vi "Layer2_TransmitAndReceiveResponse.vi"(4 "error in (no error)":errorcluster, 5 "Expecting Response":bool=TRUE, 6 "Message":string="TestStation1", 7 "Serial Port to Use":refnum<visa-resource-name>="COM8") -> (0 "Error Out":errorcluster, 1 "Response":string, 2 "Success":bool, 3 "Serial Port to Use (out)":refnum<visa-resource-name>)   [LabVIEW 2012]
uses:
  Arduino_Serial_GlobalConstants.vi
panel:
  out "Write Buffer":string
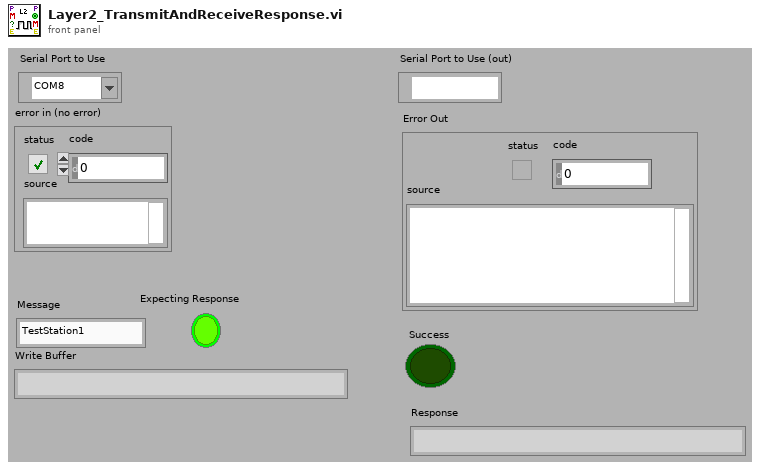
[diagram p1: front panel]
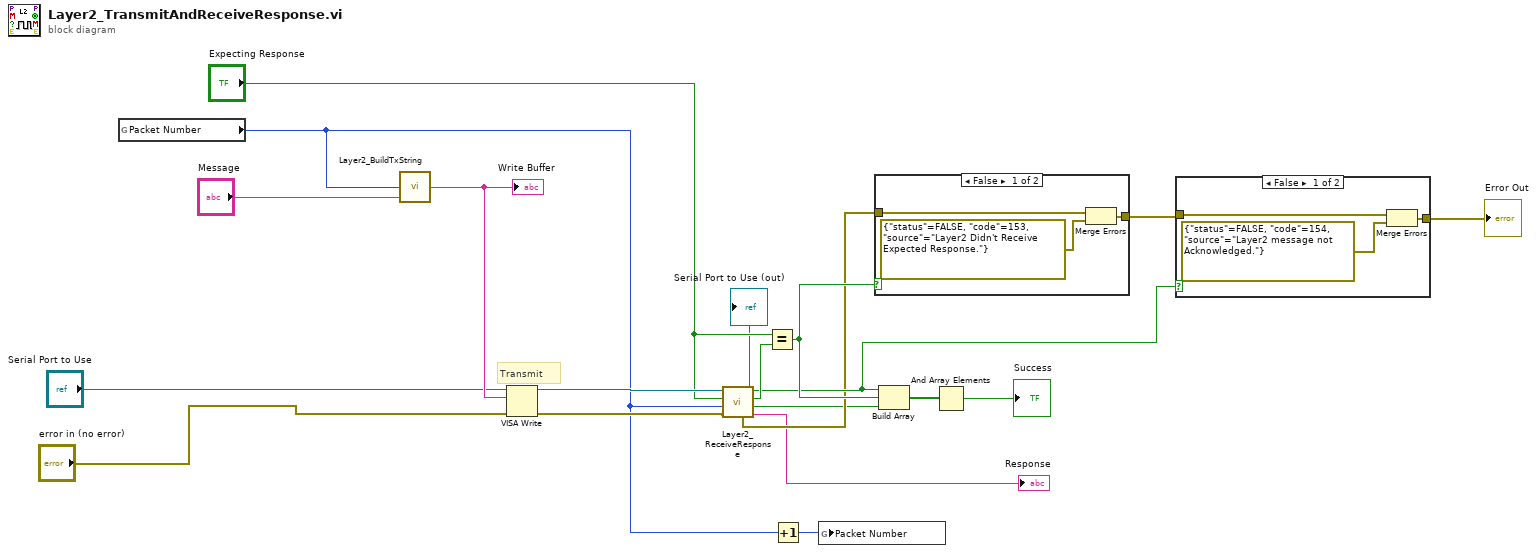
[diagram p0: block diagram]
diagram:
  # "Transmit"
  n1 = global read "Arduino_Serial_GlobalConstants.vi" "Packet Number"() -> (w11:u16)
  n2 = call "Layer2_BuildTxString.vi"("Message"="Message", "PacketNum"=w11) -> ("Write Buffer"=w17:string)  [unwired: 1 in]
  "Write Buffer" <- w17
  n3 = VISA Write(VISA resource name="Serial Port to Use", write buffer=w17, error in (no error)="error in (no error)") -> (VISA resource name out=w20:refnum<visa-resource-name>, error out=w19:errorcluster)  [unwired: 1 out]
  n4 = call "Layer2_ReceiveResponse.vi"("Error In"=w19, "PacketNum\nWaiting Ack"=w11, "Expecting Response"="Expecting Response", "Serial Port to Use"=w20) -> ("Layer2 Payload"=→"Response":string, "No Errors"=w5:bool, "Response Received"=w13:bool, "Msg Acknowledged"=w7:bool, "Error Out"=w6:errorcluster, "Serial Port to Use (out)"=→"Serial Port to Use (out)":refnum<visa-resource-name>)  [unwired: 2 in]
  n5 = Equal?(x="Expecting Response", y=w13) -> (x = y?=w10:bool)
  n6 = Increment(x=w11) -> (x+1=w14:u16)
  n7 = global write "Arduino_Serial_GlobalConstants.vi" "Packet Number"(w14) -> ()
  n8 = case shown="False" w10 {
    tunnel: w6 -> [w22 w24]
    tunnel: [w23 w24] -> w9
    frame False {
      n9 = Merge Errors(w22, errorcluster {"status"=FALSE, "code"=153, "source"="Layer2 Didn't Receive Expected Response."} ("error in")) -> (w23:errorcluster)
    }
    frame True {
    }
  }
  n10 = Build Array(w7, w10, w5) -> (w16:bool[])
  n11 = And Array Elements(Boolean array=w16) -> (logical AND=→"Success":bool)
  n12 = case shown="False" w7 {
    tunnel: w9 -> [w26 w28]
    tunnel: [w27 w28] -> w8
    frame False {
      n13 = Merge Errors(w26, errorcluster {"status"=FALSE, "code"=154, "source"="Layer2 message not Acknowledged."} ("error in")) -> (w27:errorcluster)
    }
    frame True {
    }
  }
  "Error Out" <- w8
